vi "3.2.vi"() -> ()   [LabVIEW 2017]
panel:
  in  "B":dbl
  in  "A":dbl
  out "Result":dbl
  in  "功能选择":enum16{"相除", "相乘", "相减", "相加"}(ring)
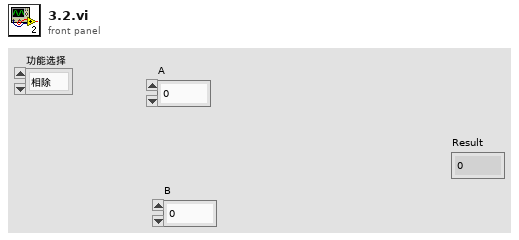
[diagram p1: front panel]
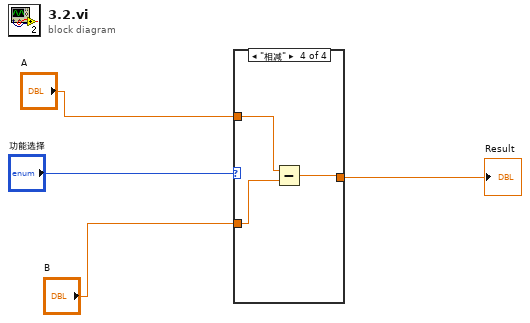
[diagram p0: block diagram]
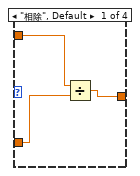
[diagram p2: hidden frame]
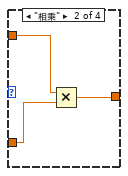
[diagram p3: hidden frame]
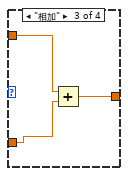
[diagram p4: hidden frame]
diagram:
  n1 = case shown="\"相减\"" "功能选择" {
    tunnel: "A" -> [w7 w8 w13 w15]
    tunnel: "B" -> [w6 w9 w12 w14]
    tunnel: [w5 w10 w11 w16] -> w1
    frame "相除", Default {
      n2 = Divide(x=w7, y=w6) -> (x/y=w5:dbl)
    }
    frame "相乘" {
      n3 = Multiply(x=w8, y=w9) -> (x*y=w10:dbl)
    }
    frame "相加" {
      n4 = Add(x=w13, y=w12) -> (x+y=w11:dbl)
    }
    frame "相减" {
      n5 = Subtract(x=w15, y=w14) -> (x-y=w16:dbl)
    }
  }
  "Result" <- w1
